vi "TestValueChange_ExplicitVIRef_ChangeCaught.vi"(8 "error in (no error)":errorcluster, 11 "TestCase in":refnum<class "TestAutoRegistration.lvclass">) -> (0 "error out":errorcluster, 3 "TestCase out":refnum<class "TestAutoRegistration.lvclass">)   [LabVIEW 2017, in "TestAutoRegistration.lvclass"]
uses:
  TestAutoRegistration.lvclass
  <vilib>/addons/_JKI Toolkits/VI Tester/TestCase.llb/TestCase.lvclass
  Source/Framework/ActorEvents/AutoRegistration/AutoRegistration.lvclass
  C:/Program Files (x86)/National Instruments/LabVIEW 2017/vi.lib/addons/_JKI Toolkits/VI Tester/TestCase.llb/TestCase.lvclass
panel:
  in  "Numeric":dbl
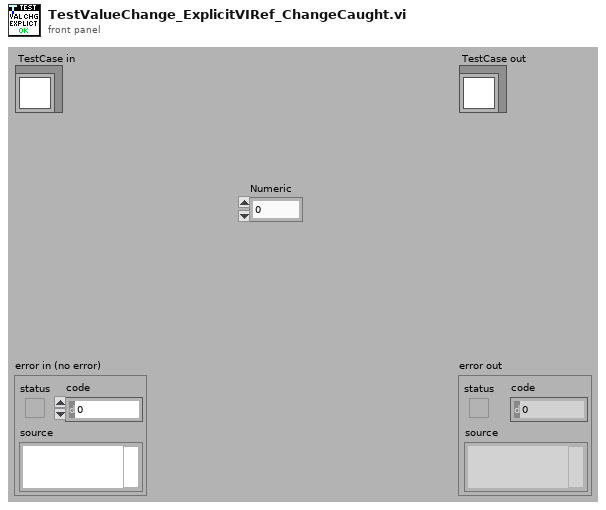
[diagram p1: front panel]
types:
  T1 = typedef "AutoRegistration.lvlib/AutoRegistration.lvclass/Auto-Event Registration Refnum.ctl" = refnum<event-registration>
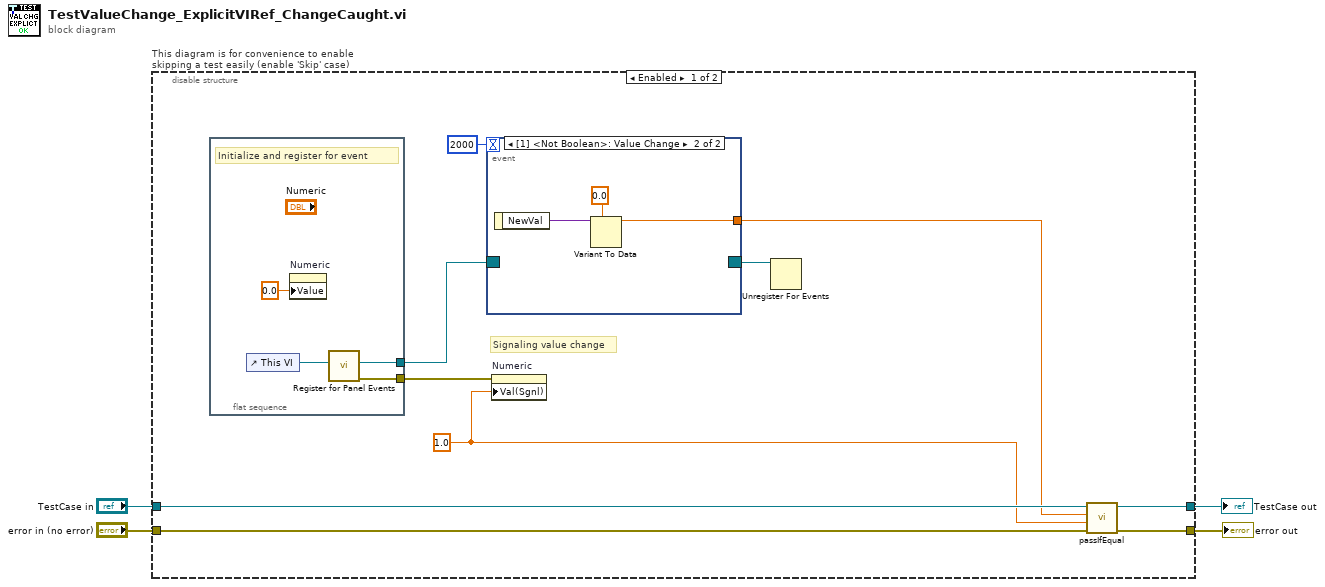
[diagram p0: block diagram]
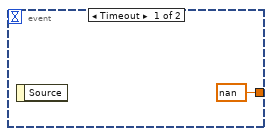
[diagram p2: hidden frame]
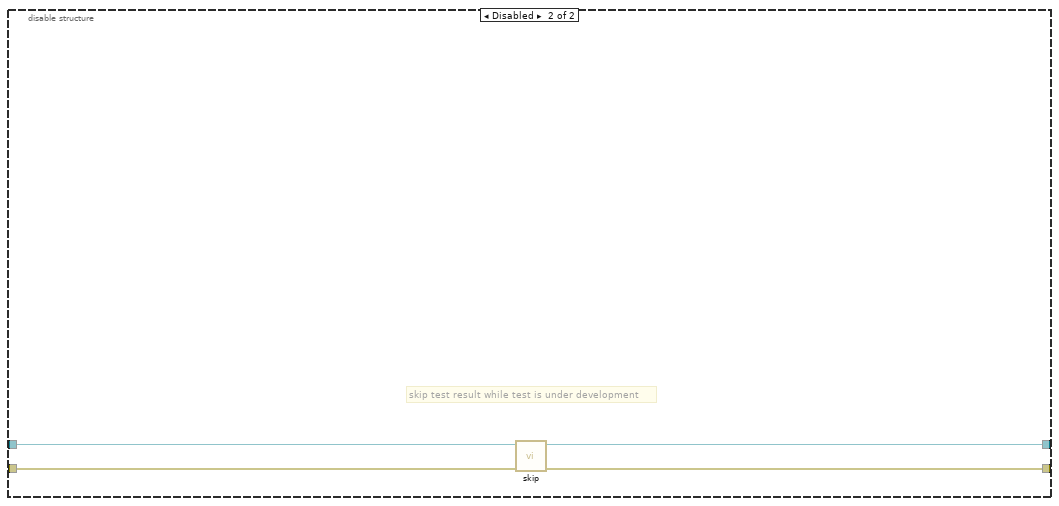
[diagram p3: hidden frame]
diagram:
  n1 = disable-structure "This diagram is for convenience to enable skipping a test easily (enable 'Skip' case)" shown="Enabled" {
    disable-tunnel: "TestCase in" -> [w14 w26]
    disable-tunnel: [w13 w24] -> w1
    disable-tunnel: [w12 w25] -> w3
    disable-tunnel: "error in (no error)" -> [w11 w23]
    frame Enabled {
      w7 = 1.0 ("Value (Signaling)")
      # "Signaling value change"
      n2 = flat-sequence {
        tunnel: [w21] -> w8
        tunnel: [w20] -> w10
        frame #0 {
          # "Initialize and register for event"
          n3 = control-ref of="This VI"() -> (w22:refnum<vi>)
          n4 = property on="Numeric" class="DigNum (strict)"("Value"=0.0 ("Value (Signaling)")) -> ()  [unwired: 2 in, 2 out]
          n5 = call "Register for Panel Events.vi"("VI Refnum (Calling VI)"=w22) -> ("error out"=w21:errorcluster, "Auto-Event Registration Refnum"=w20:T1)  [unwired: 7 in, 2 out]
        }
      }
      n6 = event shown="[1] <Not Boolean>: Value Change" {
        selector: w10 -> [_ _]
        dyn-events: [_ _] -> w6
        timeout: 2000 -> [_ _]
        tunnel: [nan ("Numeric") w16] -> w9
        event Timeout {
          n7 = event-data() -> ()  [unwired: 1 in, 1 out]
        }
        event Value Change {
          n8 = event-data() -> ("NewVal"=w18:variant)  [unwired: 1 in]
          n9 = Variant To Data(type=0.0 ("Numeric"), Variant=w18) -> (data=w16:dbl)  [unwired: 1 in, 1 out]
        }
      }
      n10 = property on="Numeric" class="DigNum (strict)"(error in=w8, "Val(Sgnl)"=w7) -> ()  [unwired: 1 in, 2 out]
      n11 = Unregister For Events(event registration refnum=w6) -> ()  [unwired: 1 in, 1 out]
      n12 = call-dynamic "passIfEqual.vi"("error in (no error)"=w11, "y"=w7, "x"=w9, "TestCase in"=w14) -> ("error out"=w12:errorcluster, "TestCase out"=w13:refnum<class "TestAutoRegistration.lvclass">)  [unwired: 6 in]
    }
    frame Disabled {
      # "skip test result while test is under development"
      n13 = call <vilib>:"skip.vi"("error in (no error)"=w23, "TestCase in"=w26) -> ("error out"=w25:errorcluster, "TestCase out"=w24:refnum<class "TestAutoRegistration.lvclass">)  [unwired: 8 in]
    }
  }
  "error out" <- w3
  "TestCase out" <- w1
